vi "Write Default Values to disk.vi"(0 "reference in":refnum<class "Generic Utilities.lvclass">, 5 "error in (no error)":errorcluster, 6 "AppData Option":T1(ring), 7 "Control Label":string, 9 "Caption":string, 11 "Value (XML String)":string) -> (14 "reference out":refnum<class "Generic Utilities.lvclass">, 19 "error out":errorcluster)   [LabVIEW 2022 SP3, in "Generic Utilities.lvclass"]
doc: "This writes an XML file with the value using XML string as data and \"Label\" and \"Caption\" to build the file name in a given application data folder."
uses:
  Generic Utilities.lvclass
  <vilib>/Utility/sysdir.llb/System Directory Type.ctl
  <vilib>/Utility/xml.llb/Write to XML File(string).vi
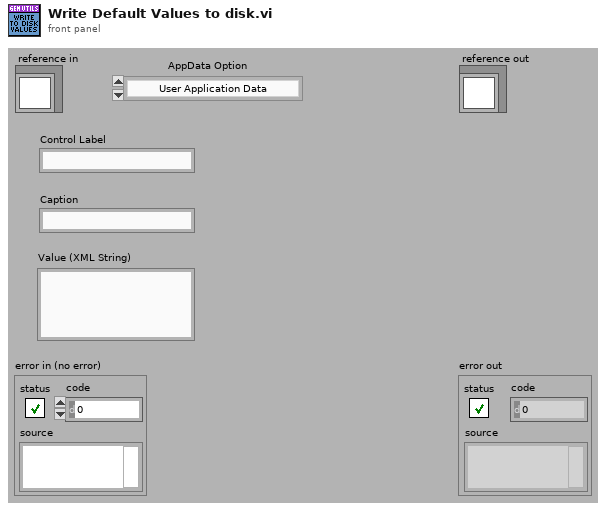
[diagram p1: front panel]
types:
  T1 = enum16{"User Application Data", "Public Application Data"}
  T2 = typedef "Generic Utilities.lvclass/ObjectAttributes.ctl" = cluster{"GUI Parameters":T3, "State Machine Control":cluster{"Timeout":i32, "State Queue":string[], "State History":string[], "State History Length":i32}, "Logging File Path":path, "OBJ not a refnum?":bool, "Timer Start":timestamp, "FP Refnums":T4}
  T3 = typedef "Generic Utilities.lvclass/GUI Parameters.ctl" = cluster{"Application Name":string, "GUI VI Ref":refnum<vi>, "Close Panel?":bool, "Message Window ref":refnum<vi>, "Version #":string}
  T4 = typedef "Generic Utilities.lvclass/FP Refnums.ctl" = cluster{"Panel refnum":refnum<vi>, "Control Labels":string[], "Refnums":refnum<vi>[]}
  T5 = typedef "System Directory Type.ctl" = i32
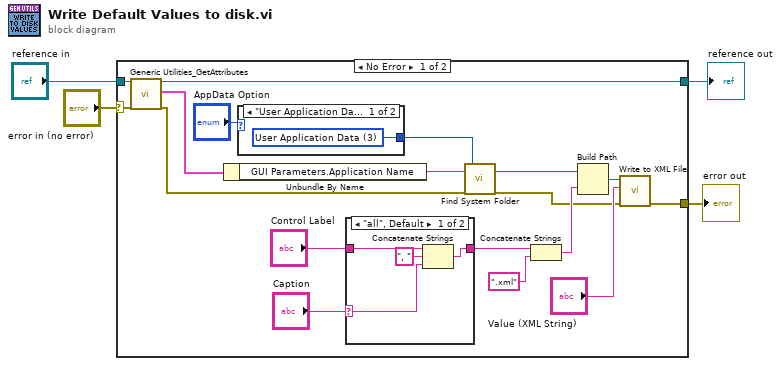
[diagram p0: block diagram]
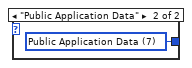
[diagram p2: hidden frame]
diagram:
  n1 = case shown="No Error" "error in (no error)" {
    selector: "error in (no error)" -> [w22 w31]
    tunnel: [w7 w31] -> w3
    tunnel: [w21 w30] -> w1
    tunnel: "reference in" -> [w19 w30]
    frame No Error {
      n2 = call "Generic Utilities_GetAttributes.vi"("reference in"=w19, "error in (no error)"=w22) -> ("reference out"=w21:refnum<class "Generic Utilities.lvclass">, "attributes"=w20:T2, "error out"=w17:errorcluster)  [unwired: 14 in, 1 out]
      n3 = Unbundle By Name(w20) -> ("GUI Parameters.Application Name"=w18:string)
      n4 = case shown="\"User Application Data\", Default" "AppData Option" {
        tunnel: [w23 w24] -> w6
        frame "User Application Data", Default {
          w23 = T5 3 items=["User Home"=0, "User Desktop"=1, "User Documents"=2, "User Application Data"=3, "User Preferences"=4, "User Temporary"=5, "Public Documents"=6, "Public Application Data"=7, "Public Preferences"=8, "Public Cache"=13, "System Core Libraries"=9, "System Installed Libraries"=10, "Application Files"=11, "Boot Volume Root"=12] ("system directory type")
        }
        frame "Public Application Data" {
          w24 = T5 7 items=["User Home"=0, "User Desktop"=1, "User Documents"=2, "User Application Data"=3, "User Preferences"=4, "User Temporary"=5, "Public Documents"=6, "Public Application Data"=7, "Public Preferences"=8, "Public Cache"=13, "System Core Libraries"=9, "System Installed Libraries"=10, "Application Files"=11, "Boot Volume Root"=12] ("system directory type")
        }
      }
      n5 = case shown="\"all\", Default" "Caption" {
        selector: "Caption" -> [w25 _]
        tunnel: [w28 w29] -> w11
        tunnel: "Control Label" -> [w27 w29]
        frame "all", Default {
          n6 = Concatenate Strings(w27, ", " ("string"), w25) -> (w28:string)
        }
        frame "" {
        }
      }
      n7 = call "Find System Folder.vi"("Application Name"=w18, "error in (no error)"=w17, "system directory type"=w6) -> ("System Folder"=w9:path, "error out"=w8:errorcluster)  [unwired: 15 in]
      n8 = Concatenate Strings(w11, ".xml" ("string")) -> (w14:string)
      n9 = Build Path(base path=w9, name or relative path=w14) -> (appended path=w16:path)
      n10 = call-poly <vilib>:"Write to XML File.vi"("error in (no error)"=w8, "XML Input"="Value (XML String)", "XML File Path"=w16) -> ("error out"=w7:errorcluster)  [unwired: 6 in, 2 out]
    }
    frame Error {
    }
  }
  "error out" <- w3
  "reference out" <- w1
